vi "EPS-Read Measurements.vi"(8 "error in":errorcluster, 11 "EPS Setting In":T2) -> (0 "error out":errorcluster, 2 "Measurement Data":T1, 3 "EPS Setting Out":T2)   [LabVIEW 2018]
uses:
  Data Def/EPS-Setting.ctl
  Data Def/EPS-Measurement Data.ctl
  Data Def/EPS-Access Mode.ctl
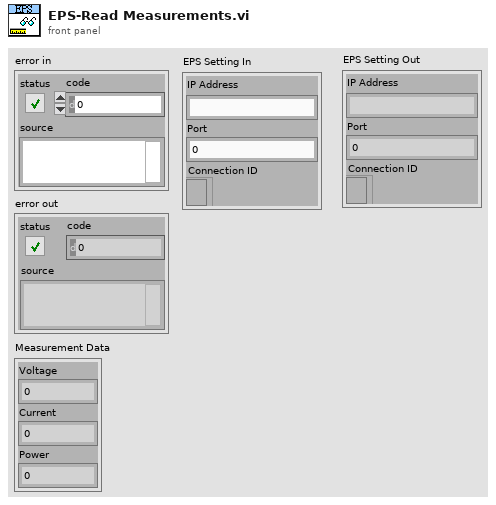
[diagram p1: front panel]
types:
  T1 = typedef "EPS-Measurement Data.ctl" = cluster{"Voltage":dbl, "Current":dbl, "Power":dbl}
  T2 = typedef "EPS-Setting.ctl" = cluster{"IP Address":string, "Port":u16, "Connection ID":refnum<k5>}
  T3 = typedef "EPS-Access Mode.ctl" = enum16{"Read", "Write"}
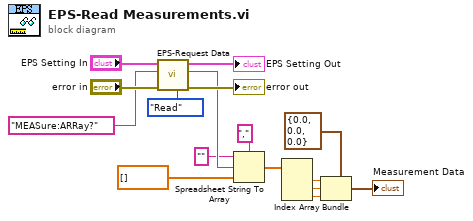
[diagram p0: block diagram]
diagram:
  n1 = call "EPS-Request Data.vi"("Access Mode"=EPS-Access_Mode."Read", "error in"="error in", "Requst Data"="MEASure:ARRay?", "EPS Setting In"="EPS Setting In") -> ("error out"=→"error out":errorcluster, "Response Data"=w10:string, "EPS Setting Out"=→"EPS Setting Out":T2)  [unwired: 5 in]
  n2 = Spreadsheet String To Array(delimiter (Tab)=",", format string="", spreadsheet string=w10, array type (2D Dbl)=dbl[] []) -> (array=w6:dbl[])
  n3 = Index Array(array=w6) -> (element #1=w5:dbl, element #2=w4:dbl, element #3=w3:dbl)  [unwired: 3 in]
  n4 = Bundle(cluster=T1 {"Voltage"=0.0, "Current"=0.0, "Power"=0.0} ("Measurement Data"), "Voltage"=w5, "Current"=w4, "Power"=w3) -> (→"Measurement Data":T1)
